vi "Resize.vi"(4 "Send events? [T]":bool=TRUE, 6 "Defer Panel Updates? [T]":bool=TRUE, 7 "VI Refnum":refnum<vi>, 8 "error in (no error)":errorcluster, 10 "Bounds":T1, 11 "MMI Scaling in":refnum<class "Interaction By Refererence.lvclass">) -> (0 "error out":errorcluster, 2 "Resized":string[](array[string]), 3 "MMI Scaling out":refnum<class "Interaction By Refererence.lvclass">)   [LabVIEW 2021, in "Interaction By Refererence.lvclass"]
uses:
  Interaction By Refererence.lvclass
  <vilib>/Utility/miscctls.llb/LVRectTypeDef.ctl
  Interaction By Refererence.lvclass/Interaction By Refererence.ctl
  IObject.lvclass
  IContainer/Interaction/Interaction.lvclass
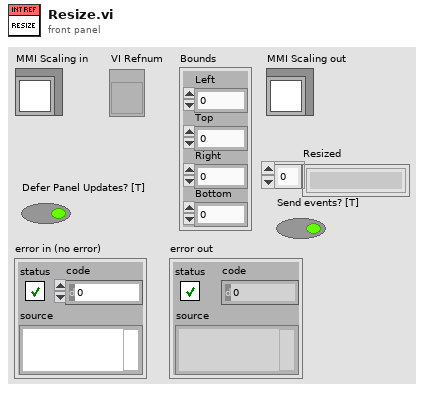
[diagram p1: front panel]
types:
  T1 = typedef "LVRectTypeDef.ctl" = cluster{"Left":i16, "Top":i16, "Right":i16, "Bottom":i16}
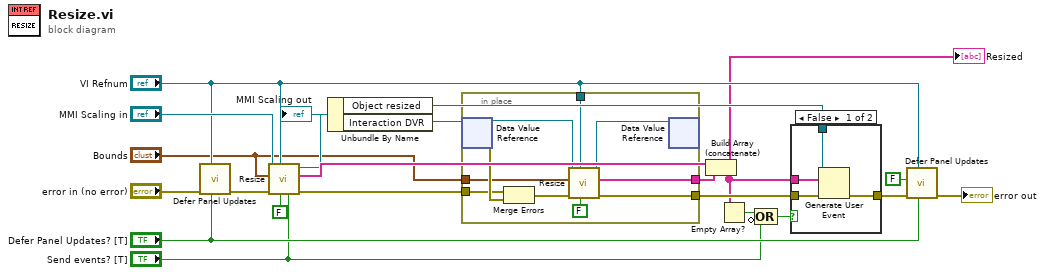
[diagram p0: block diagram]
diagram:
  n1 = call "Defer Panel Updates.vi"("Set Defer Panel Updates? [T]"="Defer Panel Updates? [T]", "VI Refnum"="VI Refnum", "error in (no error)"="error in (no error)") -> ("error out"=w15:errorcluster)  [unwired: 8 in]
  n2 = call-parent "Resize.vi"("Send events? [T]"="Send events? [T]", "Defer Panel Updates? [T]"=FALSE, "VI Refnum"="VI Refnum", "error in (no error)"=w15, "Bounds"="Bounds", "MMI Scaling in"="MMI Scaling in") -> ("error out"=w19:errorcluster, "Resized"=w18:string[], "MMI Scaling out"=w16:refnum<class "Interaction By Refererence.lvclass">)  [unwired: 3 in]
  "MMI Scaling out" <- w16
  n3 = Unbundle By Name(w16) -> ("Object resized"=w4:refnum<user-event>, "Interaction DVR"=w21:refnum<data-value>)
  n4 = in-place {
    in-place-border: [w28] -> w6
    in-place-border: w19 -> [w30]
    in-place-border: "VI Refnum" -> [w25]
    in-place-border: "Bounds" -> [w24]
    in-place-border: [w23] -> w8
    n5 = in-place-dvr #1(w21) -> (w27:refnum<class "Interaction.lvclass">, w31:errorcluster)
    n6 = Merge Errors(w30, w31) -> (w29:errorcluster)
    n7 = call-dynamic "Resize.vi"("Defer Panel Updates? [T]"=FALSE, "VI Refnum"=w25, "error in (no error)"=w29, "Bounds"=w24, "MMI Scaling in"=w27) -> ("error out"=w28:errorcluster, "Resized"=w23:string[], "MMI Scaling out"=w26:refnum<class "Interaction.lvclass">)  [unwired: 4 in]
    n8 = in-place-dvr #1(w26) -> ()  [unwired: 2 out]
  }
  n9 = Build Array (concatenate)(w18, w8) -> (w3:string[])
  "Resized" <- w3
  n10 = Empty Array?(array=w3) -> (empty?=w7:bool)
  n11 = Compound Arithmetic op=OR(w7, invert "Send events? [T]") -> (w1:bool)
  n12 = case shown="False" w1 {
    tunnel: w4 -> [w35 _]
    tunnel: [w34 w36] -> w5
    tunnel: w6 -> [w33 w36]
    tunnel: w3 -> [w32 _]
    frame False {
      n13 = Generate User Event(user event=w35, event data cluster=w32, error in=w33) -> (error out=w34:errorcluster)  [unwired: 1 in, 1 out]
    }
    frame True {
    }
  }
  n14 = call "Defer Panel Updates.vi"("Set Defer Panel Updates? [T]"="Defer Panel Updates? [T]", "VI Refnum"="VI Refnum", "error in (no error)"=w5, "Defer Panel Updates? [T]"=FALSE) -> ("error out"=→"error out":errorcluster)  [unwired: 7 in]
